vi "Keyence.FTP.Flush.vi"(8 "error in (no error)":errorcluster, 10 "host":string) -> (0 "error out":errorcluster, 3 "FTP Session out":T1)   [LabVIEW 2016]
uses:
  <vilib>/FTP/ftp0.llb/FTP Session.ctl
  <vilib>/FTP/NI_FTP.lvlib
panel:
  out "Files":string[](array[string])
  in  "remote port (21)":u16=21
  in  "password":string="admin"
  in  "user":string="admin"
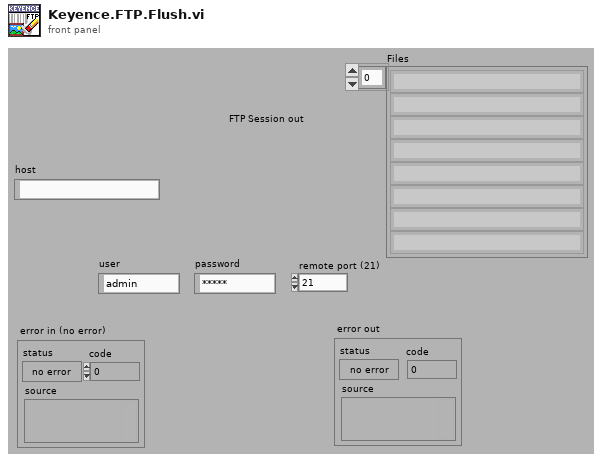
[diagram p1: front panel]
types:
  T1 = typedef "NI_FTP.lvlib/FTP Session.ctl" = refnum<k5>
  T2 = typedef "NI_FTP.lvlib/FTP File Info.ctl" = cluster{"type":enum16{"unknown", "file", "dir", "link"}, "permissions":string, "owner":string, "group":string, "size":i32, "date":string, "name":string, "link name":string}
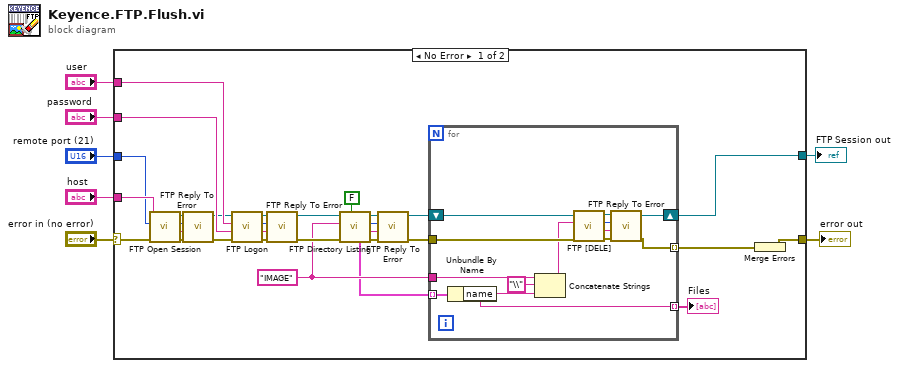
[diagram p0: block diagram]
diagram:
  n1 = case shown="No Error" "error in (no error)" {
    selector: "error in (no error)" -> [w16 w51]
    tunnel: "host" -> [w37 _]
    tunnel: "user" -> [w36 _]
    tunnel: "password" -> [w35 _]
    tunnel: "remote port (21)" -> [w24 _]
    tunnel: [w15 w51] -> w3
    tunnel: [w8 _] -> w1
    frame No Error {
      w13 = "IMAGE" ("directory path")
      n2 = call <vilib>:"FTP Open Session.vi"("error in (no error)"=w16, "remote port (21)"=w24, "address"=w37) -> ("error out"=w34:errorcluster, "reply string"=w31:string, "reply code"=w32:i32, "ftp session"=w33:T1)  [unwired: 5 in]
      n3 = call <vilib>:"FTP Reply To Error.vi"("error in (no error)"=w34, "reply string in"=w31, "reply code in"=w32, "ftp session"=w33) -> ("error out"=w29:errorcluster, "ftp session out"=w30:T1)  [unwired: 2 out]
      n4 = call <vilib>:"FTP Logon.vi"("error in (no error)"=w29, "password"=w35, "user"=w36, "ftp session"=w30) -> ("error out"=w28:errorcluster, "reply string"=w25:string, "reply code"=w26:i32, "ftp session out"=w27:T1)  [unwired: 4 in]
      n5 = call <vilib>:"FTP Reply To Error.vi"("error in (no error)"=w28, "reply string in"=w25, "reply code in"=w26, "ftp session"=w27) -> ("error out"=w17:errorcluster, "ftp session out"=w18:T1)  [unwired: 2 out]
      n6 = call <vilib>:"FTP Directory Listing.vi"("active (T)"=FALSE, "error in (no error)"=w17, "directory path"=w13, "ftp session"=w18) -> ("error out"=w22:errorcluster, "reply string"=w20:string, "reply code"=w21:i32, "ftp session out"=w23:T1, "dir list"=w12:T2[])  [unwired: 3 in]
      n7 = call <vilib>:"FTP Reply To Error.vi"("error in (no error)"=w22, "reply string in"=w20, "reply code in"=w21, "ftp session"=w23) -> ("error out"=w11:errorcluster, "ftp session out"=w10:T1)  [unwired: 2 out]
      n8 = for {
        tunnel: w11 -> [w50]
        tunnel: w12 -> [w44] mode=indexing
        tunnel: w13 -> [w43]
        tunnel: [w41] -> w14 mode=indexing
        shift-right: [w40] -> w8
        shift-left: w10 -> [w49]
        tunnel: [w38] -> w9 mode=indexing
        n9 = Unbundle By Name(w44) -> ("name"=w38:string)
        n10 = Concatenate Strings(w43, "\\" ("string"), w38) -> (w39:string)
        n11 = call <vilib>:"FTP [DELE].vi"("error in (no error)"=w50, "file path"=w39, "ftp session"=w49) -> ("error out"=w48:errorcluster, "reply string"=w45:string, "reply code"=w46:i32, "ftp session out"=w47:T1)  [unwired: 5 in]
        n12 = call <vilib>:"FTP Reply To Error.vi"("error in (no error)"=w48, "reply string in"=w45, "reply code in"=w46, "ftp session"=w47) -> ("error out"=w41:errorcluster, "ftp session out"=w40:T1)  [unwired: 2 out]
      }
      "Files" <- w9
      n13 = Merge Errors(w14) -> (w15:errorcluster)
    }
    frame Error {
    }
  }
  "error out" <- w3
  "FTP Session out" <- w1
